vi "dfd_Get Multirate FIR Params.vi"(8 "error in (no error)":errorcluster, 9 "type (FLP)":enum16{"FLP", "FXP"}(ring), 10 "alternate mode":T2=-1 items=["Default"=-1, "No Rate Change"=0, "Interpolation"=1, "Decimation"=2, "Interpolated"=3, "Rational"=4], 11 "multirate filter in":T3={"mMRate_Structure"=enum."CIC", "mMRate_Mode"=0, "mMRate_Factor"=1, "mMRate_FIRParams"={"mMRate_FIR_H"=[], "mMRate_FIR_IsNyquist?"=FALSE, "mMRate_FIR_IsSymmetric?"=FALSE}, "mMRate_CICParams"={"mMRate_CIC_#Stage"=2, "mMRate_CIC_Lag"=1, "mMRate_CIC_Type"=enum."Lowpass"}, "mMRate_Order"=1, "mMRate_Version"="1.0", "mMRate_Comments"="1.0", "mMRate_RationalFactor"={"mMRate_L"=-1, "mMRate_M"=-1}, "mMRate_Fs"=0.0, "mMRate_Quantized?"=FALSE, "mMRate_QFilterGain"=1.0, "mMRate_CoefWl"=16, "mMRate_Scaling"={"mMRate_ScaleByPowerOf2?"=FALSE, "mMRate_ScaleType"=enum."Time Domain 1-Norm"}, "mMRate_InputWl"=0, "mMRate_OutputWl"=0, "mMRate_OutputMode"=enum."Nearest", "mMRate_MultMode"=enum."Truncated", "mMRate_BitPruning"=FALSE, "mMRate_GainWl"=16, "mMRate_OutputFwl"=0, "mMRate_SumIwl"=0, "mMRate_InputIwl "=16, "mMRate_SumWl"=32, "mMRate_CoefIwl"=0} {"mMRate_SumWl" min=1 max=32 step=1; "mMRate_InputIwl" min=1 max=32 step=1; "mMRate_GainWl" min=1 max=32 step=1; "mMRate_OutputWl" min=1 max=32 step=1; "mMRate_InputWl" min=1 max=32 step=1; "mMRate_CoefWl" min=1 max=32 step=1; "mMRate_Mode" items=["Default"=-1, "No Rate Change"=0, "Interpolation"=1, "Decimation"=2, "Interpolated"=3, "Rational"=4]}) -> (0 "error out":errorcluster, 1 "mode":T2 items=["Default"=-1, "No Rate Change"=0, "Interpolation"=1, "Decimation"=2, "Interpolated"=3, "Rational"=4], 2 "factor":T1, 3 "h (n)":dbl[](array[numeric]), 4 "order":i32)   [LabVIEW 2017, in "NI_DigFilterLicensed.lvlib"]
uses:
  <vilib>/addons/Digital Filter Design/NI_DigFilterLicensed.lvlib
  <vilib>/addons/Digital Filter Design/_Objects.llb/DFD Multirate Filter Obj.ctl
  <vilib>/addons/Digital Filter Design/_Objects.llb/DFD Multirate Mode.ctl
  <vilib>/addons/Digital Filter Design/_Objects.llb/DFD Coef Norm Type.ctl
  <vilib>/addons/Digital Filter Design/_Objects.llb/DFD Round-off Mode.ctl
  <vilib>/addons/Digital Filter Design/_Objects.llb/DFD FXP MRate Multiply Mode.ctl
  <vilib>/addons/Digital Filter Design/_Objects.llb/DFD Multirate Rational Factor.ctl
  <vilib>/addons/Digital Filter Design/NI_DigFilter_FXP.lvlib
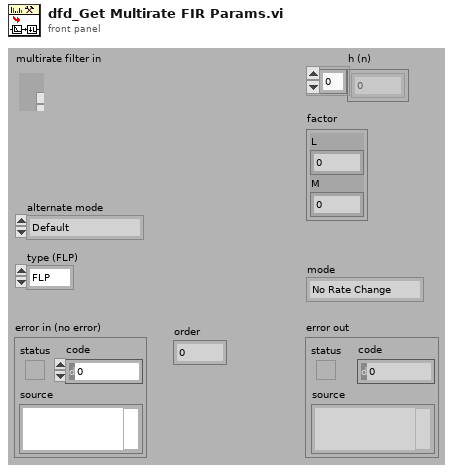
[diagram p1: front panel]
types:
  T1 = typedef "NI_DigFilterLicensed.lvlib/DFD Multirate Rational Factor.ctl" = cluster{"L":i32, "M":i32}
  T2 = typedef "NI_DigFilterLicensed.lvlib/DFD Multirate Mode.ctl" = i16
  T3 = typedef "NI_DigFilterLicensed.lvlib/DFD Multirate Filter Obj.ctl" = cluster{"mMRate_Structure":enum16{"CIC", "FIR", "IIR", "Lattice"}, "mMRate_Mode":T2, "mMRate_Factor":i32, "mMRate_FIRParams":cluster{"mMRate_FIR_H":dbl[], "mMRate_FIR_IsNyquist?":bool, "mMRate_FIR_IsSymmetric?":bool}, "mMRate_CICParams":cluster{"mMRate_CIC_#Stage":i32, "mMRate_CIC_Lag":i32, "mMRate_CIC_Type":enum16{"Lowpass", "Highpass"}}, "mMRate_Order":i32, "mMRate_Version":string, "mMRate_Comments":string, "mMRate_RationalFactor":cluster{"mMRate_L":i32, "mMRate_M":i32}, "mMRate_Fs":dbl, "mMRate_Quantized?":bool, "mMRate_QFilterGain":dbl, "mMRate_CoefWl":i16, "mMRate_Scaling":cluster{"mMRate_ScaleByPowerOf2?":bool, "mMRate_ScaleType":T4}, "mMRate_InputWl":i16, "mMRate_OutputWl":i16, "mMRate_OutputMode":T5, "mMRate_MultMode":T6, "mMRate_BitPruning":bool, "mMRate_GainWl":i16, "mMRate_OutputFwl":i16, "mMRate_SumIwl":i16, "mMRate_InputIwl ":i16, "mMRate_SumWl":i16, "mMRate_CoefIwl":i16}
  T4 = typedef "NI_DigFilterLicensed.lvlib/DFD Coef Norm Type.ctl" = enum16{"No Norm", "Time Domain 1-Norm", "Time Domain 2-Norm", "Time Domain Inf-Norm"}
  T5 = typedef "NI_DigFilterLicensed.lvlib/DFD Round-off Mode.ctl" = enum16{"Nearest", "Truncation"}
  T6 = typedef "NI_DigFilterLicensed.lvlib/DFD FXP MRate Multiply Mode.ctl" = enum16{"Truncated", "Full"}
  T7 = typedef "NI_DigFilterLicensed.lvlib/dfd_Internal Quantization Settings.ctl" = cluster{"source":T8, "wl":i16, "iwl":i16, "overflow mode":enum16{"Saturation", "Wrap"}, "rounding mode":enum16{"Nearest", "Truncation"}, "signed?":bool}
  T8 = typedef "NI_DigFilterLicensed.lvlib/dfd_Internal Quantization Srcs.ctl" = u16
  T9 = typedef "NI_DigFilterLicensed.lvlib/DFD Quantization Settings.ctl" = cluster{"source":T10, "wl":i16, "iwl":i16, "overflow mode":enum16{"Saturation", "Wrap"}, "rounding mode":enum16{"Nearest", "Truncation"}, "signed?":bool}
  T10 = typedef "NI_DigFilterLicensed.lvlib/DFD Quantization Sources.ctl" = u16
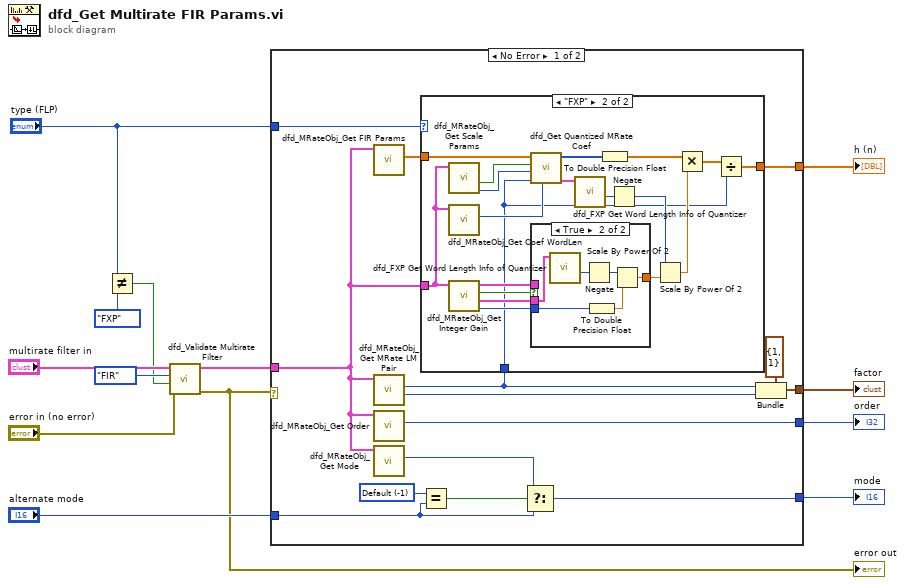
[diagram p0: block diagram]
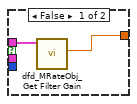
[diagram p3: hidden frame]
diagram:
  n1 = Not Equal?(x="type (FLP)", y=enum16{"FLP", "FXP"}."FXP" ("x")) -> (x != y?=w2:bool)
  n2 = call <vilib>:"dfd_Validate Multirate Filter.vi"("error in (no error)"="error in (no error)", "skip FXP? (T)"=w2, "preferred structure"=enum16{"CIC", "FIR", "IIR", "Lattice"}."FIR" ("structure"), "multirate filter in"="multirate filter in") -> ("error out"=w1:errorcluster, "multirate filter out"=w3:T3)  [unwired: 6 out]
  "error out" <- w1
  n3 = case shown="No Error" w1 {
    tunnel: w3 -> [w15 _]
    tunnel: [w24 _] -> w10
    tunnel: [w26 _] -> w9
    tunnel: [w21 _] -> w7
    tunnel: "alternate mode" -> [w16 _]
    tunnel: [w20 _] -> w6
    tunnel: "type (FLP)" -> [w23 _]
    frame No Error {
      w25 = T2 -1 items=["Default"=-1, "No Rate Change"=0, "Interpolation"=1, "Decimation"=2, "Interpolated"=3, "Rational"=4] ("alternate mode")
      n4 = call <vilib>:"dfd_MRateObj_Get FIR Params.vi"("multirate filter in"=w15) -> ("h(n)"=w22:dbl[])  [unwired: 10 out]
      n5 = call <vilib>:"dfd_MRateObj_Get MRate LM Pair.vi"("multirate filter in"=w15) -> ("M"=w18:i32, "L"=w14:i32)  [unwired: 1 in, 8 out]
      n6 = call <vilib>:"dfd_MRateObj_Get Order.vi"("multirate filter in"=w15) -> ("order"=w21:i32)  [unwired: 10 out]
      n7 = call <vilib>:"dfd_MRateObj_Get Mode.vi"("multirate filter in"=w15) -> ("mode"=w17:T2)  [unwired: 10 out]
      n8 = case shown="\"FXP\"" w23 {
        tunnel: w22 -> [w28 w47]
        tunnel: [w28 w30] -> w24
        tunnel: w15 -> [_ w46]
        tunnel: w14 -> [_ w29]
        frame "FLP", Default {
        }
        frame "FXP" {
          n9 = call <vilib>:"dfd_MRateObj_Get Scale Params.vi"("multirate filter in"=w46) -> ("scale type"=w44:T4, "scale by Power of 2?"=w45:bool)  [unwired: 9 out]
          n10 = call <vilib>:"dfd_MRateObj_Get Coef WordLen.vi"("multirate filter in"=w46) -> ("coef wl"=w43:i16)  [unwired: 10 out]
          n11 = call <vilib>:"dfd_MRateObj_Get Integer Gain.vi"("multirate filter"=w46) -> ("I32 gain"=w41:i32, "Gain quantizer"=w40:T7, "on FPGA?"=w42:bool, "dup multirate filter"=w39:T3)  [unwired: 7 out]
          n12 = call <vilib>:"dfd_Get Quantized MRate Coef.vi"("coef wl"=w43, "L"=w29, "scale type"=w44, "scale by Power of 2?"=w45, "h"=w47) -> ("coef quantizer"=w36:T9, "h (I32)"=w37:i32[])  [unwired: 5 out]
          n13 = case shown="True" w42 {
            tunnel: w41 -> [_ w53]
            tunnel: w40 -> [_ w51]
            tunnel: [w48 w50] -> w35
            tunnel: w39 -> [w49 _]
            frame False {
              n14 = call <vilib>:"dfd_MRateObj_Get Filter Gain.vi"("multirate filter in"=w49) -> ("gain"=w48:dbl)  [unwired: 10 out]
            }
            frame True {
              n15 = call <vilib>:"dfd_FXP Get Word Length Info of Quantizer.vi"("quantization settings"=w51) -> ("fwl"=w54:i16)  [unwired: 10 out]
              n16 = Negate(x=w54) -> (-x=w55:i16)
              n17 = To Double Precision Float(number=w53) -> (double precision float=w52:dbl)
              n18 = Scale By Power Of 2(n=w55, x=w52) -> (x*2^n=w50:dbl)
            }
          }
          n19 = call <vilib>:"dfd_FXP Get Word Length Info of Quantizer.vi"("quantization settings"=w36) -> ("fwl"=w38:i16)  [unwired: 10 out]
          n20 = To Double Precision Float(number=w37) -> (double precision float=w33:dbl[])
          n21 = Negate(x=w38) -> (-x=w34:i16)
          n22 = Scale By Power Of 2(n=w34, x=w35) -> (x*2^n=w32:dbl)
          n23 = Multiply(x=w33, y=w32) -> (x*y=w31:dbl[])
          n24 = Divide(x=w31, y=w29) -> (x/y=w30:dbl[])
        }
      }
      n25 = Equal?(x=w25, y=w16) -> (x = y?=w27:bool)
      n26 = Select(t=w17, s=w27, f=w16) -> (s? t:f=w26:T2)
      n27 = Bundle(cluster=T1 {"L"=1, "M"=1} ("rational factor"), "L"=w14, "M"=w18) -> (w20:T1)
    }
    frame Error {
    }
  }
  "h (n)" <- w10
  "mode" <- w9
  "order" <- w7
  "factor" <- w6
